vi "RavenDAQ.vi"() -> ()   [LabVIEW 2013]
uses:
  <vilib>/Analysis/NI_AALBase.lvlib
  <vilib>/Analysis/NI_AALPro.lvlib
panel:
  out "Hit Map":bool
  out "Acquisition":bool
  out "Spectrum acquisition":bool
  in  "Timestamp number":i32=12
  out "Stop collecting 2":bool
  out "Packages String":u16[](array[numeric])
  out "Packeges Array":u16[][](array[numeric])
  out "Rate (Hz)":i32
  out "Rate2":dbl(knob) scale=1500.0..30000.0
  out "Rate 2":dbl(knob) scale=10.0..2000.0
  in  "Stop collecting":bool
  in  "milliseconds to wait":u32
  in  "Number of APVs":i32=2
  in  "Max packet size (9016 jumbo)":i32=9016
  in  "Listen IP (10.0.0.2)":string="10.0.0.3"
  in  "Port (6006)":u16=6006
  out "Pedestal acquisition":bool
  out "Fast analysis":bool
  out "Raw data viewer":bool
  out "Latency scan":bool
  out "Collecting data":bool
  in  "Tab Control":T1(tab)
  in  "Raw data viewer":bool
  out "Raw Data":u16[](graph)
  out "Array":i32[][](array[numeric]) format="%x"
  out "APV":i32 format="%x"
  in  "Filename":string
  out "Event saved":i32
  in  "Saving data":bool
  in  "Path":path
  out "Saving":bool
  in  "Latency scan mode":bool
  in  "Control APV":i8
  out "APV number 2":u8
  in  "Min":i32=2100
  in  "Max":i32=2500
  out "Good event 2":i32
  out "data out 3":u16[](graph)
  out "Good event":bool
  out "Rate good event (Hz)":i32
  in  "Tab Control 2":enum32{"Pedestal", "Spectrum", "Hit Map"}(tab)
  in  "Show pad N":i32
  out "Mean":dbl format="%0.2f"
  out "Standard deviation":dbl format="%0.2f"
  in  "Pedestal acquisition":bool
  in  "RESET pedestals":bool
  out "Mean on":i32[](array[numeric])
  out "128 Channel Sum Histogram":T2(graph)
  in  "Spectrum acquisition":bool
  in  "RESET data":bool
  in  "Target pad":i32
  in  "Sigma cut":i32=4
  in  "Head and tail cut":i32=2
  out "Hit count":i32
  out "Energy distribution":dbl[][](graph)
  out "Hit position":i32[](graph)
  out "Rate good event (Hz)":i32
  out "Intensity Graph":i32[][](graph)
  in  "Hit Map":bool
  in  "Mapping file":path
  in  "Triggered data saver":bool
  in  "Path":path
  in  "Filename":string
  out "Saved events":i32
  out "Saver":bool
  out "Rate good event (Hz)  2":i32
  in  "Fast Analysis":bool
  in  "Analyze APV":u8
  in  "Digital 1 threshold":i32=1450
  in  "Digital 0 threshold":i32=2950
  out "N received event":i32=3649
  # "INFN Trieste                                     Marco Baruzzo elbaru90@gmail.com"
  # "Before take a pedestal!!!!!!!!"
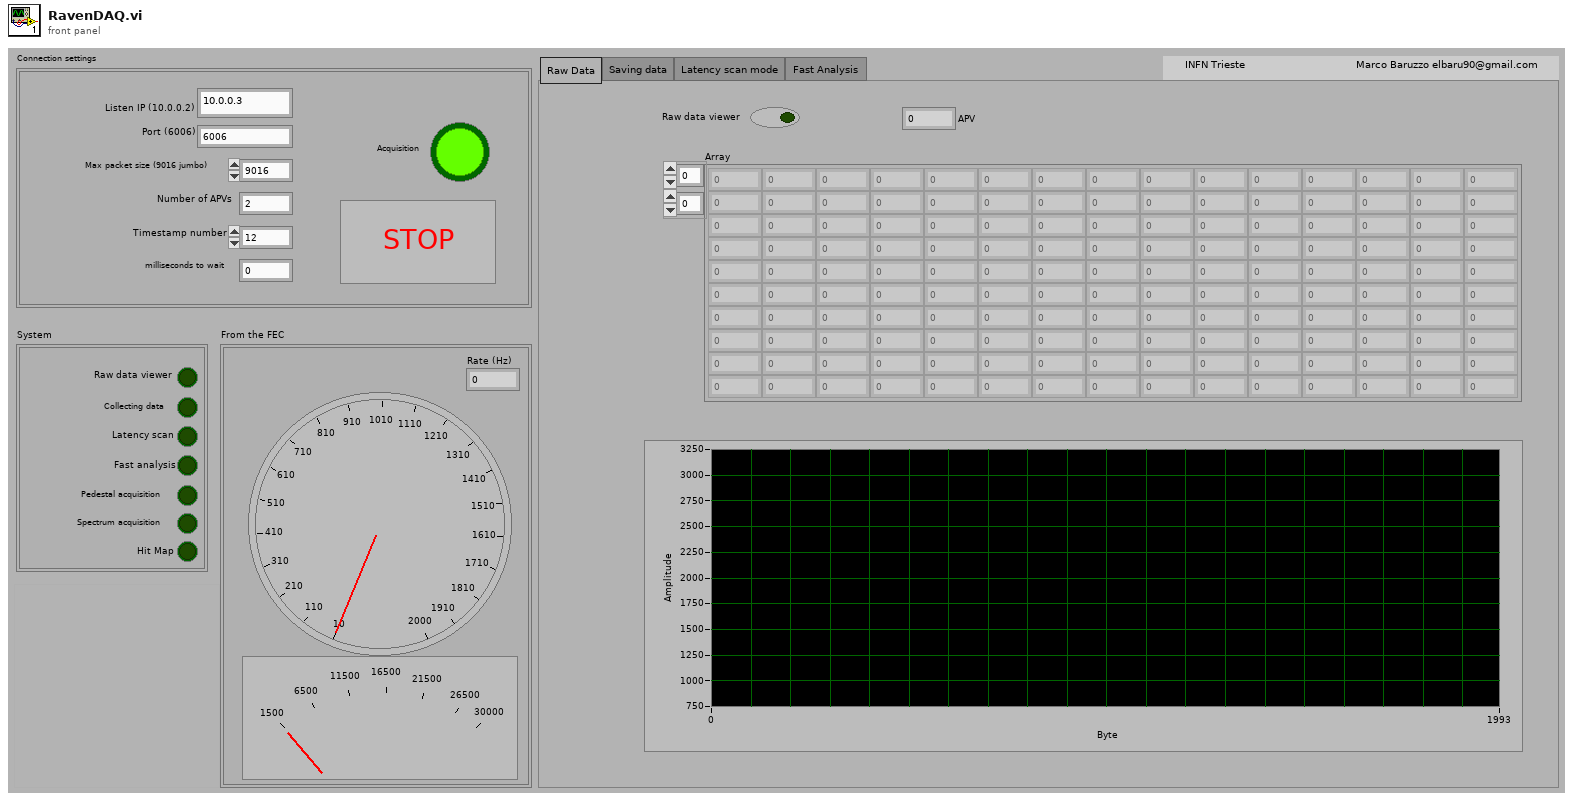
[diagram p1: front panel]
types:
  T1 = enum32{"Raw Data", "Saving data", "Latency scan mode", "Fast Analysis "}
  T2 = cluster{"X Values":dbl[], "Histogram: h(x)":i32[]}
  T3 = enum16{"open", "replace", "create", "open or create", "replace or create", "replace or create with confirmation"}
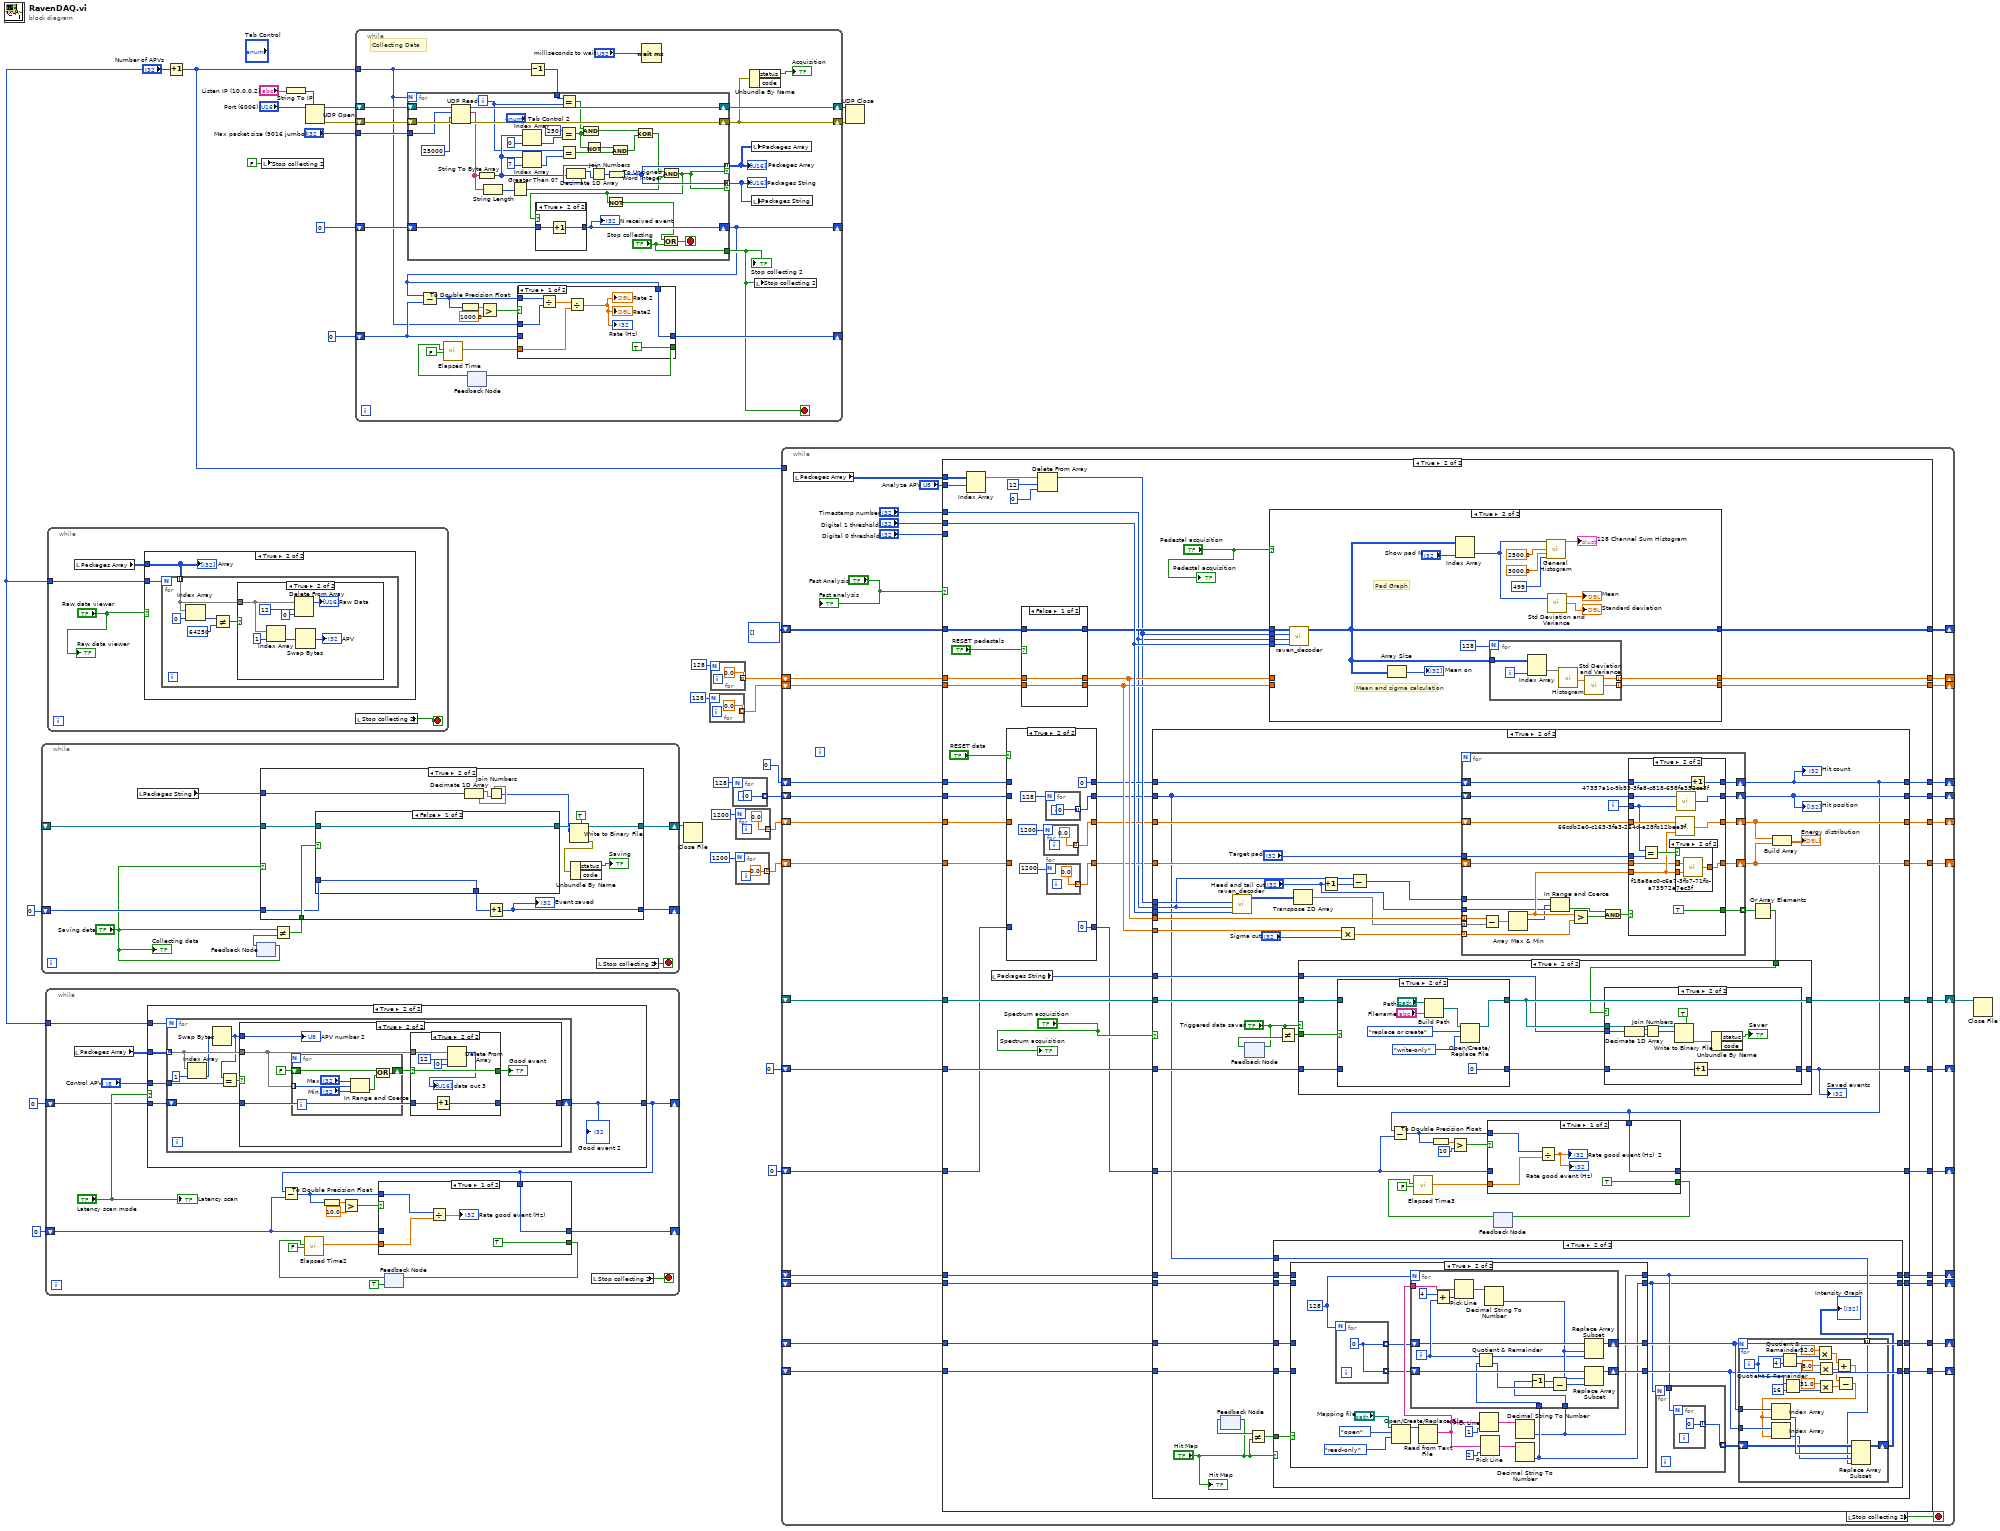
[diagram p0: block diagram]
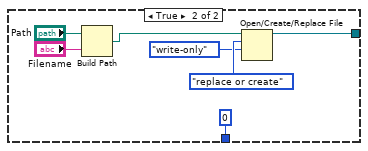
[diagram p5: hidden frame]
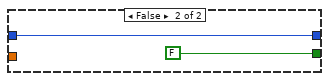
[diagram p6: hidden frame]
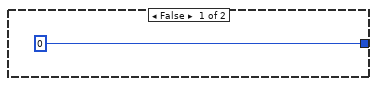
[diagram p7: hidden frame]
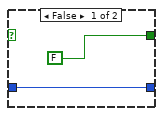
[diagram p9: hidden frame]
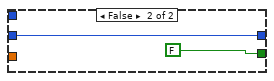
[diagram p10: hidden frame]
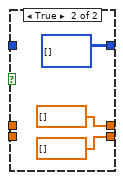
[diagram p14: hidden frame]
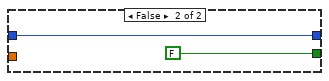
[diagram p16: hidden frame]
diagram:
  n1 = while {
    shift-right: [w38] -> _
    shift-left: 0 -> [w40]
    shift-right: [w39] -> w10
    shift-left: _ -> [w37]
    stop <- w33 stop-if-true
    n2 = local read "Packages String"() -> (w36:u16[])
    n3 = feedback #1() -> (w35:bool)  [unwired: 1 in]
    n4 = feedback-in #1("Saving data") -> ()
    n5 = Not Equal?(x="Saving data", y=w35) -> (x != y?=w41:bool)
    n6 = case shown="True" "Saving data" {
      tunnel: [w43 w54] -> w38
      tunnel: w40 -> [w43 w47]
      tunnel: w37 -> [w42 w55]
      tunnel: [w42 w57] -> w39
      tunnel: w36 -> [_ w53]
      tunnel: w41 -> [_ w48]
      frame False {
      }
      frame True {
        n7 = case shown="False" w48 {
          tunnel: [w59 w65] -> w56
          tunnel: w55 -> [w59 _]
          tunnel: w47 -> [w58 _]
          tunnel: [w58 0] -> w46
          frame False {
          }
          frame True {
            n8 = Build Path(base path="Path", name or relative path="Filename") -> (appended path=w61:path)
            n9 = Open/Create/Replace File(file path (use dialog)=w61, operation (0:open)=T3."replace or create", access (0:read/write)=enum16{"read/write", "read-only", "write-only"}."write-only") -> (refnum out=w65:refnum<file>)  [unwired: 3 in, 2 out]
          }
        }
        n10 = Decimate 1D Array(w53) -> (w52:u16[], w51:u16[])
        n11 = Join Numbers(hi=w51, lo=w52) -> ((hi.lo)=w50:u32[])
        n12 = Increment(x=w46) -> (x+1=w54:i32)
        "Event saved" <- w54
        n13 = Write to Binary File(file (use dialog)=w56, data=w50, 5:TRUE ("prepend array or string size? (T)")) -> (refnum out=w57:refnum<file>, error out=w44:errorcluster)  [unwired: 3 in, 1 out]
        n14 = Unbundle By Name(w44) -> ("status"=→"Saving":bool)  [unwired: 1 out]
      }
    }
    n15 = local read "Stop collecting 2"() -> (w33:bool)
    "Collecting data" <- "Saving data"
  }
  n16 = Increment(x="Number of APVs") -> (x+1=w9:i32)
  n17 = while {
    tunnel: w9 -> [w83]
    shift-right: [w70] -> _
    shift-left: 0 -> [w82]
    shift-right: [w71] -> _
    shift-left: 0 -> [w69]
    stop <- w79 stop-if-true
    n18 = local read "Packeges Array"() -> (w80:u16[][])
    n19 = case shown="True" "Latency scan mode" {
      tunnel: w83 -> [_ w97]
      tunnel: "Control APV" -> [_ w96]
      tunnel: [0 w95] -> w70
      tunnel: w82 -> [_ w94]
      tunnel: w80 -> [_ w93]
      frame False {
      }
      frame True {
        n20 = for {
          N: w97 -> [_]
          tunnel: w96 -> [w104]
          shift-right: [w102] -> w95
          shift-left: w94 -> [w101]
          tunnel: w93 -> [w100] mode=indexing
          n21 = Index Array(array=w100, index=1 ("ch id")) -> (element=w99:u16)
          n22 = Swap Bytes(anything=w99) -> (byte swapped=w98:u16)
          n23 = Equal?(x=w98, y=w104) -> (x = y?=w103:bool)
          n24 = case shown="True" w103 {
            tunnel: w100 -> [_ w108]
            tunnel: [w106 w109] -> w102
            tunnel: w101 -> [w106 w110]
            tunnel: w98 -> [_ w107]
            frame False {
            }
            frame True {
              n25 = for {
                tunnel: w108 -> [w126] mode=indexing
                shift-right: [w123] -> w112
                shift-left: FALSE -> [w125]
                n26 = In Range and Coerce(upper limit="Max", x=w126, lower limit="Min") -> (In Range?=w124:bool)  [unwired: 1 out]
                n27 = Or(x=w125, y=w124) -> (x .or. y?=w123:bool)
              }
              n28 = case shown="True" w112 {
                selector: w112 -> [_ w122]
                tunnel: [FALSE w122] -> w111
                tunnel: w110 -> [w114 w121]
                tunnel: [w114 w120] -> w109
                tunnel: w108 -> [_ w117]
                frame False {
                }
                frame True {
                  n29 = Increment(x=w121) -> (x+1=w120:i32)
                  n30 = Delete From Array(array=w117, length=12, index=0) -> (array with subset deleted=→"data out 3":u16[])  [unwired: 1 out]
                }
              }
              "Good event" <- w111
              "APV number 2" <- w107
            }
          }
        }
        "Good event 2" <- w95
      }
    }
    n31 = Subtract(x=w70, y=w69) -> (x-y=w74:i32)
    n32 = To Double Precision Float(number=w74) -> (double precision float=w73:dbl)
    n33 = Greater?(x=w73, y=10.0) -> (0:w75:bool)
    n34 = feedback #2(TRUE) -> (w72:bool)
    n35 = call "Elapsed Time2"("Reset"=w72, "Auto Reset"=FALSE) -> ("Elapsed Time (s)"=w76:dbl)  [unwired: 10 in, 7 out]
    n36 = case shown="True" w75 {
      tunnel: w69 -> [_ w90]
      tunnel: w74 -> [w86 _]
      tunnel: w76 -> [w89 _]
      tunnel: [TRUE FALSE] -> w68
      tunnel: [w87 w90] -> w71
      tunnel: w70 -> [w87 _]
      frame True {
        n37 = Divide(x=w86, y=w89) -> (x/y=→"Rate good event (Hz)":dbl)
      }
      frame False {
      }
    }
    n38 = feedback-in #2(w68) -> ()
    n39 = local read "Stop collecting 2"() -> (w79:bool)
    "Latency scan" <- "Latency scan mode"
  }
  n40 = while {
    tunnel: w9 -> [w131]
    stop <- w129 stop-if-true
    n41 = local read "Packeges Array"() -> (w130:u16[][])
    n42 = case shown="True" "Raw data viewer" {
      tunnel: w131 -> [_ w134]
      tunnel: w130 -> [_ w133]
      frame False {
      }
      frame True {
        n43 = for {
          N: w134 -> [_]
          tunnel: w133 -> [w138] mode=indexing
          n44 = Index Array(array=w138, index=0) -> (element=w137:u16)
          n45 = Not Equal?(x=w137, y=64250) -> (x != y?=w136:bool)
          n46 = case shown="True" w136 {
            tunnel: w138 -> [_ w146]
            frame False {
            }
            frame True {
              n47 = Index Array(array=w146, index=1) -> (element=w144:u16)
              n48 = Delete From Array(array=w146, length=12, index=0) -> (array with subset deleted=→"Raw Data":u16[])  [unwired: 1 out]
              n49 = Swap Bytes(anything=w144) -> (byte swapped=→"APV":u16)
            }
          }
        }
        "Array" <- w133
      }
    }
    n50 = local read "Stop collecting 2"() -> (w129:bool)
    "Raw data viewer" <- "Raw data viewer"
  }
  n51 = local write "Stop collecting 2"(FALSE ("Stop collecting 2")) -> ()
  n52 = String To IP(1:"Listen IP (10.0.0.2)") -> (0:w31:u32)
  n53 = UDP Open(7:w31, 11:"Port (6006)") -> (port=w18:refnum<k16>, 0:w17:errorcluster)  [unwired: 3 in, 1 out]
  n54 = while {
    shift-right: [w156] -> _
    shift-left: 0 -> [w157]
    shift-right: [w164] -> w19
    shift-left: w18 -> [w162]
    shift-right: [w147] -> w20
    shift-left: w17 -> [w161]
    shift-right: [w151] -> _
    shift-left: 0 -> [w160]
    tunnel: "Max packet size (9016 jumbo)" -> [w159]
    tunnel: w9 -> [w150]
    stop <- w153 stop-if-true
    # "Collecting Data"
    n55 = feedback #3() -> (w170:bool)  [unwired: 1 in]
    n56 = call "Elapsed Time"("Reset"=w170, "Auto Reset"=FALSE) -> ("Elapsed Time (s)"=w167:dbl)  [unwired: 10 in, 7 out]
    n57 = Decrement(x=w150) -> (x-1=w149:i32)
    n58 = for {
      N: w150 -> [_]
      shift-right: [w205] -> w147
      shift-left: w161 -> [w212]
      shift-right: [w204] -> w164
      shift-left: w162 -> [w213]
      shift-right: [w209] -> w151
      shift-left: w160 -> [w210]
      tunnel: ["Stop collecting"] -> w153
      tunnel: [w203] -> w163 mode=indexing if=w180
      tunnel: [w203] -> w158 mode=concatenating if=w180
      tunnel: w159 -> [w202]
      tunnel: w149 -> [w193]
      i -> [w188]
      stop <- w196 stop-if-true
      n59 = UDP Read(connection ID=w213, max size (548)=w202, timeout ms (25000)=25000, 8:w212) -> (data out=w198:string, error out=w205:errorcluster, 3:w204:refnum<k16>)  [unwired: 2 out]
      n60 = String To Byte Array(string=w198) -> (unsigned byte array=w195:u8[])
      n61 = String Length(string=w198) -> (length=w211:i32)
      n62 = Greater Than 0?(x=w211) -> (x > 0?=w199:bool)
      n63 = Index Array(array=w195, index=0) -> (element=w192:u8)
      n64 = Index Array(array=w195, index=7 ("ch id")) -> (element=w189:u8)
      n65 = Equal?(x=u8 250, y=w192) -> (x = y?=w184:bool)
      n66 = Equal?(x=w193, y=w188) -> (x = y?=w190:bool)
      n67 = Equal?(x=w188, y=w189) -> (x = y?=w183:bool)
      n68 = Decimate 1D Array(w195) -> (w207:u8[], w206:u8[])
      n69 = And(x=w190, y=w184) -> (x .and. y?=w187:bool)
      n70 = Not(x=w184) -> (.not. x?=w182:bool)
      n71 = Join Numbers(hi=w206, lo=w207) -> ((hi.lo)=w208:u16[])
      n72 = To Unsigned Word Integer(number=w208) -> (unsigned 16bit integer=w203:u16[])
      n73 = And(x=w182, y=w183) -> (x .and. y?=w181:bool)
      n74 = Exclusive Or(1:w181, 2:w187) -> (0:w186:bool)
      n75 = And(x=w186, y=w199) -> (x .and. y?=w180:bool)
      n76 = case shown="True" w180 {
        tunnel: w210 -> [w214 w216]
        tunnel: [w214 w215] -> w209
        frame False {
        }
        frame True {
          n77 = Increment(x=w216) -> (x+1=w215:i32)
        }
      }
      "N received event" <- w209
      n78 = Not(x=w180) -> (.not. x?=w185:bool)
      n79 = Or(x=w185, y="Stop collecting") -> (x .or. y?=w196:bool)
    }
    "Packeges Array" <- w163
    "Packages String" <- w158
    "Stop collecting 2" <- w153
    n80 = Subtract(x=w151, y=w157) -> (x-y=w155:i32)
    n81 = To Double Precision Float(number=w155) -> (double precision float=w154:dbl)
    n82 = Greater?(x=w154, y=1000.0) -> (0:w166:bool)
    n83 = case shown="True" w166 {
      tunnel: w157 -> [_ w178]
      tunnel: w155 -> [w172 _]
      tunnel: w167 -> [w175 _]
      tunnel: [TRUE FALSE] -> w165
      tunnel: [w171 w178] -> w156
      tunnel: w150 -> [w173 _]
      tunnel: w151 -> [w171 _]
      frame True {
        n84 = Divide(x=w172, y=w173) -> (x/y=w176:dbl)
        n85 = Divide(x=w176, y=w175) -> (x/y=→"Rate 2" →"Rate2" →"Rate (Hz)":dbl)
      }
      frame False {
      }
    }
    n86 = feedback-in #3(w165) -> ()
    n87 = Wait (ms)(milliseconds to wait="milliseconds to wait") -> ()  [unwired: 1 out]
    n88 = Unbundle By Name(w147) -> ("status"=→"Acquisition":bool)  [unwired: 1 out]
    n89 = local write "Packages String"(w158) -> ()
    n90 = local write "Packeges Array"(w163) -> ()
    n91 = local write "Stop collecting 2"(w153) -> ()
  }
  n92 = Close File(refnum=w10) -> ()  [unwired: 1 in, 2 out]
  n93 = for {
    N: 128 -> [_]
    tunnel: [0.0] -> w6 mode=indexing
  }
  n94 = for {
    N: 128 -> [_]
    tunnel: [0.0] -> w4 mode=indexing
  }
  n95 = for {
    N: 128 -> [_]
    tunnel: [0] -> w26 mode=indexing
  }
  n96 = for {
    N: 1200 -> [_]
    tunnel: [0.0] -> w23 mode=indexing
  }
  n97 = for {
    N: 1200 -> [_]
    tunnel: [0.0] -> w25 mode=indexing
  }
  n98 = while {
    shift-right: [w252] -> _
    shift-left: i32[][] [] -> [w246]
    shift-right: [w251] -> _
    shift-left: w26 -> [w242]
    shift-right: [w250] -> _
    shift-left: w4 -> [w245]
    shift-right: [w249] -> _
    shift-left: w6 -> [w244]
    shift-right: [w248] -> _
    shift-left: w25 -> [w241]
    shift-right: [w247] -> _
    shift-left: 0 -> [w243]
    shift-right: [w240] -> _
    shift-left: w23 -> [w239]
    shift-right: [w233] -> w22
    shift-left: _ -> [w238]
    shift-right: [w232] -> _
    shift-left: 0 -> [w237]
    tunnel: w9 -> [_]
    shift-right: [w231] -> _
    shift-left: _ -> [w229]
    shift-right: [w230] -> _
    shift-left: _ -> [w228]
    shift-right: [w226] -> _
    shift-left: _ -> [w224]
    shift-right: [w227] -> _
    shift-left: _ -> [w225]
    shift-right: [w222] -> _
    shift-left: 0 -> [w223]
    stop <- w236 stop-if-true
    n99 = local read "Packeges Array"() -> (w235:u16[][])
    n100 = case shown="True" "Fast Analysis" {
      tunnel: "Analyze APV" -> [_ w290]
      tunnel: "Digital 1 threshold" -> [_ w319]
      tunnel: "Timestamp number" -> [_ w288]
      tunnel: w246 -> [w270 w318]
      tunnel: [w270 w289] -> w252
      tunnel: w242 -> [w269 w317]
      tunnel: [w269 w316] -> w251
      tunnel: [w268 w312] -> w250
      tunnel: w245 -> [w268 w314]
      tunnel: w244 -> [w267 w313]
      tunnel: [w267 w315] -> w249
      tunnel: [w266 w311] -> w248
      tunnel: w241 -> [w266 w310]
      tunnel: [w265 w309] -> w247
      tunnel: w243 -> [w265 w308]
      tunnel: w235 -> [_ w307]
      tunnel: [w264 w306] -> w240
      tunnel: w239 -> [w264 w305]
      tunnel: w238 -> [w262 w284]
      tunnel: w237 -> [w263 w286]
      tunnel: "Digital 0 threshold" -> [_ _]
      tunnel: [w262 w283] -> w233
      tunnel: [w263 w282] -> w232
      tunnel: [w261 w281] -> w231
      tunnel: [w260 w280] -> w230
      tunnel: w229 -> [w261 w279]
      tunnel: w228 -> [w260 w278]
      tunnel: [w259 w277] -> w227
      tunnel: [w258 w276] -> w226
      tunnel: w225 -> [w259 w275]
      tunnel: w224 -> [w258 w274]
      tunnel: w223 -> [w257 w272]
      tunnel: [w257 w273] -> w222
      frame False {
      }
      frame True {
        n101 = Index Array(array=w307, index (row)=w290) -> (element=w291:u16[])  [unwired: 1 in]
        n102 = local read "Packages String"() -> (w285:u16[])
        n103 = case shown="True" "RESET data" {
          tunnel: [w322 w330] -> w296
          tunnel: [w323 w329] -> w295
          tunnel: [w324 0] -> w294
          tunnel: w308 -> [w324 _]
          tunnel: w317 -> [w323 _]
          tunnel: w310 -> [w322 _]
          tunnel: w305 -> [w321 _]
          tunnel: [w321 w327] -> w292
          tunnel: w272 -> [w320 _]
          tunnel: [w320 0] -> w271
          frame False {
          }
          frame True {
            n104 = for {
              N: 1200 -> [_]
              tunnel: [0.0] -> w330 mode=indexing
            }
            n105 = for {
              N: 128 -> [_]
              tunnel: [0] -> w329 mode=indexing
            }
            n106 = for {
              N: 1200 -> [_]
              tunnel: [0.0] -> w327 mode=indexing
            }
          }
        }
        n107 = case shown="False" "RESET pedestals" {
          tunnel: w318 -> [w338 _]
          tunnel: [w338 i32[][] []] -> w303
          tunnel: [w337 dbl[] []] -> w302
          tunnel: [w336 dbl[] []] -> w301
          tunnel: w314 -> [w337 _]
          tunnel: w313 -> [w336 _]
          frame False {
          }
          frame True {
          }
        }
        n108 = Delete From Array(array=w291, length=12, index=0) -> (array with subset deleted=w297:u16[])  [unwired: 1 out]
        n109 = case shown="True" "Spectrum acquisition" {
          tunnel: w319 -> [_ w397]
          tunnel: w297 -> [_ w398]
          tunnel: w295 -> [w352 w364]
          tunnel: [w352 w405] -> w316
          tunnel: w302 -> [_ w395]
          tunnel: w301 -> [_ w404]
          tunnel: w296 -> [w351 w403]
          tunnel: [w351 w402] -> w311
          tunnel: [w350 w354] -> w309
          tunnel: w294 -> [w350 w401]
          tunnel: [w349 w400] -> w306
          tunnel: w292 -> [w349 w399]
          tunnel: w285 -> [_ w378]
          tunnel: w288 -> [_ w388]
          tunnel: w286 -> [w347 w382]
          tunnel: w284 -> [w348 w381]
          tunnel: [w348 w380] -> w283
          tunnel: [w347 w379] -> w282
          tunnel: [w346 w372] -> w281
          tunnel: [w345 w371] -> w280
          tunnel: w279 -> [w346 w370]
          tunnel: w278 -> [w345 w369]
          tunnel: [w344 w368] -> w277
          tunnel: [w343 w367] -> w276
          tunnel: w275 -> [w344 w366]
          tunnel: w274 -> [w343 w365]
          tunnel: w271 -> [w342 w355]
          tunnel: [w342 w356] -> w273
          frame False {
          }
          frame True {
            n110 = feedback #4() -> (w375:bool)  [unwired: 1 in]
            n111 = feedback-in #4("Hit Map") -> ()
            n112 = call "raven_decoder.vi"("Packeges Array"=w398, "Timestamp number"=w388, "Digital 1 threshold"=w397) -> ("Array (Time vs Pad) Out"=w396:u16[][])  [unwired: 7 in]
            n113 = feedback #5() -> (w384:bool)  [unwired: 1 in]
            n114 = feedback-in #5("Triggered data saver") -> ()
            n115 = Not Equal?(x=w375, y="Hit Map") -> (x != y?=w373:bool)
            n116 = case shown="True" "Hit Map" {
              tunnel: w373 -> [_ w428]
              tunnel: [w416 w419] -> w372
              tunnel: [w415 w418] -> w371
              tunnel: w370 -> [w416 w427]
              tunnel: w369 -> [w415 w426]
              tunnel: [w414 w422] -> w368
              tunnel: [w413 w421] -> w367
              tunnel: w366 -> [w414 w425]
              tunnel: w365 -> [w413 w424]
              tunnel: w364 -> [_ w423]
              frame False {
              }
              frame True {
                n117 = case shown="True" w428 {
                  tunnel: [w456 w457] -> w419
                  tunnel: [w455 w458] -> w418
                  tunnel: w427 -> [w456 _]
                  tunnel: w426 -> [w455 _]
                  tunnel: [w454 w463] -> w422
                  tunnel: [w453 w462] -> w421
                  tunnel: w425 -> [w454 _]
                  tunnel: w424 -> [w453 _]
                  frame False {
                  }
                  frame True {
                    w461 = 128
                    n118 = for {
                      N: w461 -> [_]
                      tunnel: [w473] -> w460 mode=indexing
                      tunnel: [w473] -> w459 mode=indexing
                      w473 = 0
                    }
                    n119 = Open/Create/Replace File(file path (use dialog)="Mapping file", operation (0:open)=T3."open", access (0:read/write)=enum16{"read/write", "read-only", "write-only"}."read-only") -> (refnum out=w469:refnum<file>)  [unwired: 3 in, 2 out]
                    n120 = Read from Text File(file (use dialog)=w469) -> (text=w464:string)  [unwired: 3 in, 3 out]
                    n121 = Pick Line(multi-line string=w464, line index=1) -> (output string=w466:string)  [unwired: 1 in]
                    n122 = Pick Line(multi-line string=w464, line index=2) -> (output string=w465:string)  [unwired: 1 in]
                    n123 = Decimal String To Number(string=w466) -> (number=w457:i32)  [unwired: 2 in, 1 out]
                    n124 = Decimal String To Number(string=w465) -> (number=w458:i32)  [unwired: 2 in, 1 out]
                    n125 = for {
                      N: w461 -> [_]
                      tunnel: w464 -> [w488]
                      tunnel: w458 -> [w478]
                      shift-right: [w483] -> w463
                      shift-left: w460 -> [w481]
                      shift-right: [w484] -> w462
                      shift-left: w459 -> [w482]
                      tunnel: w457 -> [w474]
                      i -> [w485]
                      n126 = Add(x=4, y=w485) -> (x+y=w487:i32)
                      n127 = Pick Line(multi-line string=w488, line index=w487) -> (output string=w486:string)  [unwired: 1 in]
                      n128 = Quotient & Remainder(x=w485, y=w478) -> (x-y*floor(x/y)=w479:i32, floor(x/y)=w477:i32)
                      n129 = Decimal String To Number(string=w486) -> (number=w480:i32)  [unwired: 2 in, 1 out]
                      n130 = Decrement(x=w474) -> (x-1=w476:i32)
                      n131 = Subtract(x=w476, y=w477) -> (x-y=w475:i32)
                      n132 = Replace Array Subset(array=w481, new element=w479, index=w480) -> (w483:i32[])
                      n133 = Replace Array Subset(array=w482, new element=w475, index=w480) -> (w484:i32[])
                    }
                  }
                }
                n134 = for {
                  N: w418 -> [_]
                  tunnel: [w430] -> w420 mode=indexing
                  tunnel: w419 -> [w429]
                  n135 = for {
                    N: w429 -> [_]
                    tunnel: [0] -> w430 mode=indexing
                  }
                }
                n136 = for {
                  tunnel: w423 -> [w434] mode=indexing
                  tunnel: w422 -> [w452]
                  tunnel: w421 -> [w451]
                  shift-right: [w450] -> w417
                  shift-left: w420 -> [w448]
                  i -> [w433]
                  n137 = Quotient & Remainder(x=w433, y=i16 4) -> (x-y*floor(x/y)=w441:i32, floor(x/y)=w442:i32)
                  n138 = Quotient & Remainder(x=w433, y=i16 16) -> (floor(x/y)=w446:i32)  [unwired: 1 out]
                  n139 = Multiply(x=32.0, y=w441) -> (x*y=w443:dbl)
                  n140 = Multiply(x=8.0, y=w442) -> (x*y=w444:dbl)
                  n141 = Multiply(x=31.0, y=w446) -> (x*y=w445:dbl)
                  n142 = Add(x=w443, y=w444) -> (x+y=w435:dbl)
                  n143 = Subtract(x=w435, y=w445) -> (x-y=w432:dbl)
                  n144 = Index Array(array=w452, index=w432) -> (element=w449:i32)
                  n145 = Index Array(array=w451, index=w432) -> (element=w447:i32)
                  n146 = Replace Array Subset(array=w448, new element=w434, index (row)=w449, index (col)=w447) -> (w450:i32[][])
                }
                "Intensity Graph" <- w417
              }
            }
            n147 = Not Equal?(x="Triggered data saver", y=w384) -> (x != y?=w385:bool)
            n148 = Transpose 2D Array(2D array=w396) -> (transposed array=w392:u16[][])
            n149 = Increment(x="Head and tail cut") -> (x+1=w390:i32)
            n150 = Multiply(x=w404, y="Sigma cut") -> (x*y=w394:dbl[])
            n151 = Subtract(x=w388, y=w390) -> (x-y=w387:i32)
            n152 = for {
              tunnel: w392 -> [w521] mode=indexing
              tunnel: w394 -> [w541] mode=indexing
              shift-right: [w540] -> w405
              shift-left: w364 -> [w538]
              shift-right: [w537] -> w402
              shift-left: w403 -> [w539]
              shift-right: [w535] -> w354
              shift-left: w401 -> [w532]
              tunnel: w387 -> [w530]
              shift-right: [w527] -> w400
              shift-left: w399 -> [w528]
              tunnel: "Target pad" -> [w529]
              tunnel: "Head and tail cut" -> [w526]
              tunnel: [w525] -> w376 mode=indexing
              tunnel: w395 -> [w522] mode=indexing
              i -> [w523]
              n153 = Subtract(x=w522, y=w521) -> (x-y=w520:dbl[])
              n154 = Array Max & Min(array=w520) -> (max value=w536:dbl, max index (indices)=w524:i32)  [unwired: 2 out]
              n155 = In Range and Coerce(upper limit=w530, x=w524, lower limit=w526) -> (In Range?=w531:bool)  [unwired: 1 out]
              n156 = Greater?(x=w536, y=w541) -> (0:w533:bool)
              n157 = And(x=w531, y=w533) -> (x .and. y?=w534:bool)
              n158 = case shown="True" w534 {
                tunnel: w538 -> [w546 w556]
                tunnel: [w546 w555] -> w540
                tunnel: w536 -> [_ w551]
                tunnel: w539 -> [w545 w557]
                tunnel: [w545 w554] -> w537
                tunnel: w532 -> [w544 w559]
                tunnel: [w544 w558] -> w535
                tunnel: w529 -> [_ w553]
                tunnel: w528 -> [w543 w550]
                tunnel: [w543 w549] -> w527
                tunnel: [FALSE TRUE] -> w525
                tunnel: w523 -> [_ w547]
                frame False {
                }
                frame True {
                  n159 = Equal?(x=w547, y=w553) -> (x = y?=w552:bool)
                  n160 = call "66cdb2e0-c163-3fe3-264d-a28fb12bee3f.vi"("index"=w551, "array in"=w557) -> ("array out"=w554:dbl[])
                  n161 = case shown="True" w552 {
                    tunnel: w551 -> [_ w563]
                    tunnel: w550 -> [w560 w562]
                    tunnel: [w560 w561] -> w549
                    frame False {
                    }
                    frame True {
                      n162 = call "f18a8ac0-c6a7-3fb7-71fb-a73972e7ec3f.vi"("index"=w563, "array in"=w562) -> ("array out"=w561:dbl[])
                    }
                  }
                  n163 = call "47357a1c-9b93-3fe8-c818-658fe352ce3f.vi"("index"=w547, "array in"=w556) -> ("array out"=w555:i32[])
                  n164 = Increment(x=w559) -> (x+1=w558:i32)
                }
              }
            }
            "Hit count" <- w354
            "Hit position" <- w405
            n165 = Subtract(x=w354, y=w355) -> (x-y=w361:i32)
            n166 = To Double Precision Float(number=w361) -> (double precision float=w360:dbl)
            n167 = Greater?(x=w360, y=10) -> (0:w362:bool)
            n168 = feedback #6() -> (w359:bool)  [unwired: 1 in]
            n169 = call "Elapsed Time3"("Reset"=w359, "Auto Reset"=FALSE) -> ("Elapsed Time (s)"=w363:dbl)  [unwired: 10 in, 7 out]
            n170 = case shown="True" w362 {
              tunnel: w355 -> [_ w411]
              tunnel: w361 -> [w407 _]
              tunnel: w363 -> [w410 _]
              tunnel: [TRUE FALSE] -> w353
              tunnel: [w408 w411] -> w356
              tunnel: w354 -> [w408 _]
              frame True {
                n171 = Divide(x=w407, y=w410) -> (x/y=→"Rate good event (Hz)  2" →"Rate good event (Hz)":dbl)
              }
              frame False {
              }
            }
            n172 = feedback-in #6(w353) -> ()
            n173 = Or Array Elements(Boolean array=w376) -> (logical OR=w377:bool)
            n174 = case shown="True" "Triggered data saver" {
              tunnel: w385 -> [_ w499]
              tunnel: w382 -> [w491 w498]
              tunnel: [w491 w492] -> w379
              tunnel: w381 -> [w490 w497]
              tunnel: [w490 w496] -> w380
              tunnel: w378 -> [_ w495]
              tunnel: w377 -> [_ w494]
              frame False {
              }
              frame True {
                n175 = case shown="True" w499 {
                  tunnel: [w511 w517] -> w496
                  tunnel: w498 -> [w512 _]
                  tunnel: [w512 0] -> w493
                  tunnel: w497 -> [w511 _]
                  frame False {
                  }
                  frame True {
                    n176 = Build Path(base path="Path", name or relative path="Filename") -> (appended path=w513:path)
                    n177 = Open/Create/Replace File(file path (use dialog)=w513, operation (0:open)=T3."replace or create", access (0:read/write)=enum16{"read/write", "read-only", "write-only"}."write-only") -> (refnum out=w517:refnum<file>)  [unwired: 3 in, 2 out]
                  }
                }
                n178 = case shown="True" w494 {
                  tunnel: w495 -> [_ w508]
                  tunnel: w496 -> [_ w504]
                  tunnel: [w500 w501] -> w492
                  tunnel: w493 -> [w500 w502]
                  frame False {
                  }
                  frame True {
                    n179 = Decimate 1D Array(w508) -> (w510:u16[], w509:u16[])
                    n180 = Join Numbers(hi=w509, lo=w510) -> ((hi.lo)=w505:u32[])
                    n181 = Write to Binary File(file (use dialog)=w504, data=w505, 5:TRUE ("prepend array or string size? (T)")) -> (error out=w507:errorcluster)  [unwired: 3 in, 2 out]
                    n182 = Increment(x=w502) -> (x+1=w501:i32)
                    n183 = Unbundle By Name(w507) -> ("status"=→"Saver":bool)  [unwired: 1 out]
                  }
                }
              }
            }
            "Saved events" <- w379
            n184 = Build Array(w402, w400) -> (→"Energy distribution":dbl[][])
            "Hit Map" <- "Hit Map"
          }
        }
        n185 = case shown="True" "Pedestal acquisition" {
          tunnel: w297 -> [_ w582]
          tunnel: w319 -> [_ w580]
          tunnel: w303 -> [w566 w569]
          tunnel: w288 -> [_ w581]
          tunnel: [w564 w568] -> w315
          tunnel: [w565 w583] -> w312
          tunnel: w302 -> [w565 _]
          tunnel: w301 -> [w564 _]
          tunnel: [w566 w567] -> w289
          frame False {
          }
          frame True {
            # "Pad Graph"
            # "Mean and sigma calculation"
            n186 = call "raven_decoder.vi"("Array (Time vs Pad) In"=w569, "Packeges Array"=w582, "Timestamp number"=w581, "Digital 1 threshold"=w580) -> ("Array (Time vs Pad) Out"=w567:u16[][])  [unwired: 6 in]
            n187 = Array Size(array=w567) -> (size(s)=→"Mean on":i32[])
            n188 = Index Array(array=w567, index (col)="Show pad N") -> (element=w571:u16[])  [unwired: 1 in]
            n189 = for {
              N: 128 -> [_]
              tunnel: [w589] -> w583 mode=indexing
              tunnel: [w588] -> w568 mode=indexing
              tunnel: w567 -> [w585]
              i -> [w584]
              n190 = Index Array(array=w585, index (col)=w584) -> (element=w587:u16[])  [unwired: 1 in]
              n191 = call <vilib>:"Histogram.vi"("X"=w587) -> ("X Values"=w586:dbl[])  [unwired: 7 in, 3 out]
              n192 = call <vilib>:"Std Deviation and Variance.vi"("X"=w586) -> ("mean"=w589:dbl, "standard deviation"=w588:dbl)  [unwired: 1 in, 1 out]
            }
            n193 = call <vilib>:"General Histogram.vi"("X"=w571, "max"=2500.0, "min"=3000.0, "# bins"=499) -> ("Histogram Graph"=→"128 Channel Sum Histogram":T2)  [unwired: 7 in, 4 out]
            n194 = call <vilib>:"Std Deviation and Variance.vi"("X"=w571) -> ("mean"=→"Mean":dbl, "standard deviation"=→"Standard deviation":dbl)  [unwired: 1 in, 1 out]
          }
        }
        "Pedestal acquisition" <- "Pedestal acquisition"
        "Spectrum acquisition" <- "Spectrum acquisition"
      }
    }
    n195 = local read "Stop collecting 2"() -> (w236:bool)
    "Fast analysis" <- "Fast Analysis"
  }
  n196 = UDP Close(connection ID=w19, 8:w20) -> ()  [unwired: 2 out]
  n197 = Close File(refnum=w22) -> ()  [unwired: 1 in, 2 out]
